vi "Destroy Timer.vi"(4 "error in (no error)":errorcluster, 7 "timer":T1) -> (0 "error out":errorcluster, 3 "timer name":string)   [LabVIEW 2011]
doc: "Destroys the specified timer. All Wait on Timer VIs that are currently waiting on this timer will time out immediately and return an error.\n\n© Copyright 1999\nCal-Bay Systems, Inc.\nwritten by James Kring"
uses:
  Timer Refnum.ctl
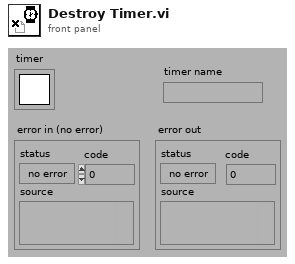
[diagram p1: front panel]
types:
  T1 = typedef "Timer Refnum.ctl" = refnum<k1>
  T2 = enum16{"open ref", "lookup ref", "close ref", "test ref", "start", "stop", "wait", "reset", "increment # waiting", "decrement #waiting"}
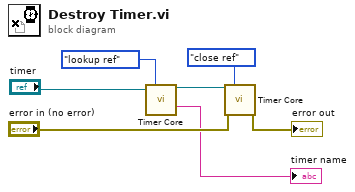
[diagram p0: block diagram]
diagram:
  n1 = call "Timer Core.vi"("timer"="timer", "function"=T2."lookup ref") -> ("timer out"=w1:T1, "name out"=→"timer name":string)  [unwired: 7 in, 5 out]
  n2 = call "Timer Core.vi"("timer"=w1, "function"=T2."close ref", "error in (no error)"="error in (no error)") -> ("error out"=→"error out":errorcluster)  [unwired: 6 in, 6 out]
